vi "svm.vi"(1 "Ch_sel":string, 2 "Repeat_train":string, 3 "Opt_met":string, 4 "Max_p":string, 5 "Rem_meth":string, 6 "Prop":string, 7 "LabVIEW Web Service Request":refnum<class "Web Request.lvclass">) -> (8 "svm_models":string, 11 "svm_training_progress":string)   [LabVIEW 2020]
uses:
  Global 1.vi
  <vilib>/wsapi/Web Request.lvclass
panel:
  # "Use the Web Service Request input terminal to call the VIs on the Web Services palette. Do not remove it from the connector pane unless you don't need access to the palette."
  # "Each additional control wired to the connector pane will be available as an input in the URL. To include an indicator in terminal-mode output (the default setting), it must also be wired to the connector pane."
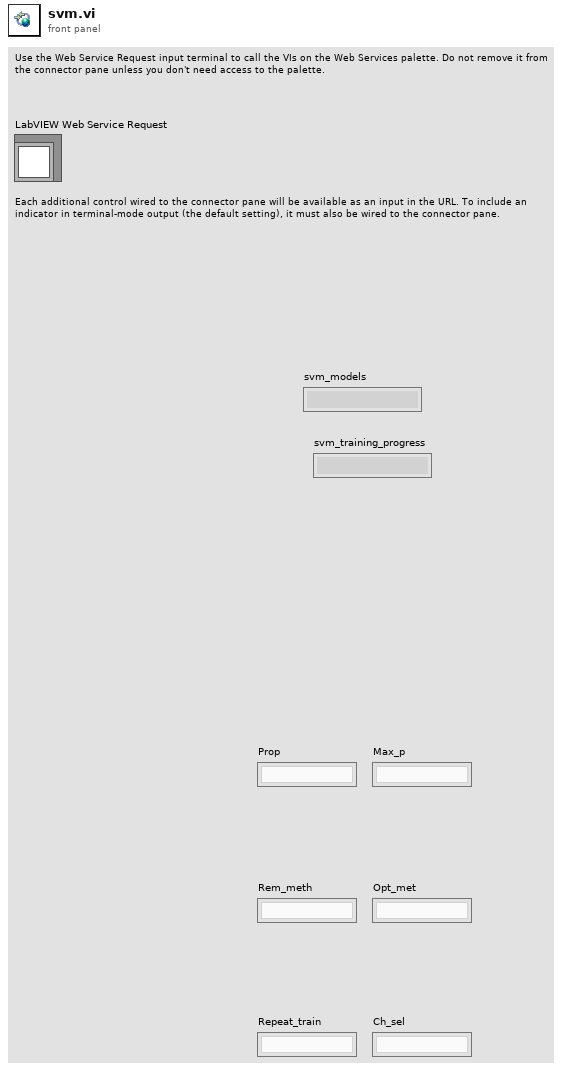
[diagram p1: front panel]
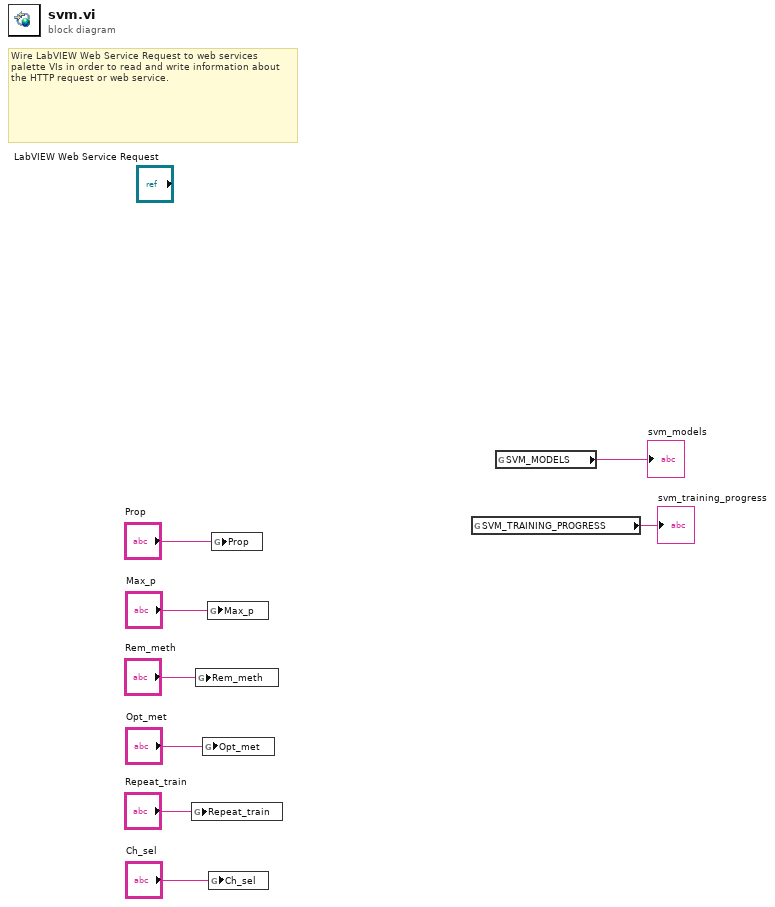
[diagram p0: block diagram]
diagram:
  # "Wire LabVIEW Web Service Request to web services palette VIs in order to read and write information about the HTTP request or web service."
  n1 = global write "Global 1.vi" "Repeat_train"("Repeat_train") -> ()
  n2 = global write "Global 1.vi" "Rem_meth"("Rem_meth") -> ()
  n3 = global write "Global 1.vi" "Opt_met"("Opt_met") -> ()
  n4 = global write "Global 1.vi" "Max_p"("Max_p") -> ()
  n5 = global write "Global 1.vi" "Ch_sel"("Ch_sel") -> ()
  n6 = global write "Global 1.vi" "Prop"("Prop") -> ()
  n7 = global read "Global 1.vi" "SVM_TRAINING_PROGRESS"() -> (→"svm_training_progress":string)
  n8 = global read "Global 1.vi" "SVM_MODELS"() -> (→"svm_models":string)
